vi "Earliest MultiFrameStructure Diagram UID.vi"(8 "error in (no error)":errorcluster, 11 "MFS ref in":refnum<vi>) -> (0 "error out":errorcluster, 1 "TLD?":bool, 2 "UID":i32, 3 "MFS ref out":refnum<vi>)   [LabVIEW 2019]
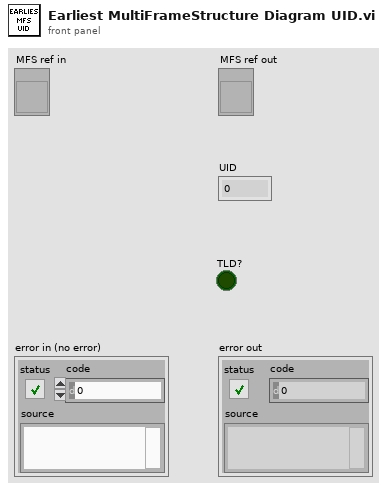
[diagram p1: front panel]
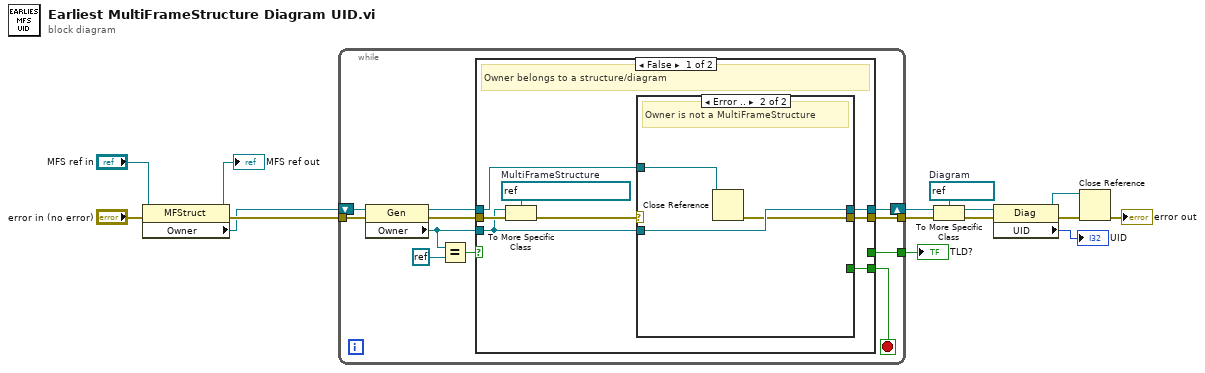
[diagram p0: block diagram]
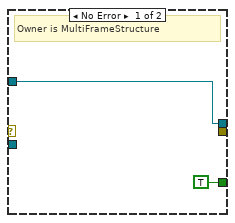
[diagram p2: hidden frame]
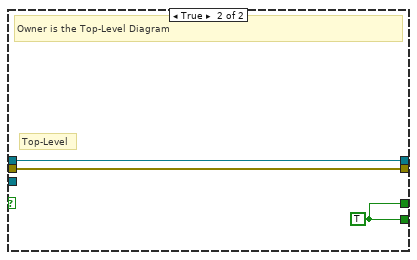
[diagram p3: hidden frame]
diagram:
  w6 = refnum<vi> refnum  # Diagram
  n1 = property class="MFStruct"(reference="MFS ref in", error in="error in (no error)") -> (reference out=→"MFS ref out":refnum<vi>, error out=w12:errorcluster, "Owner"=w11:refnum<vi>)
  n2 = while {
    tunnel: [w21] -> w7
    tunnel: w12 -> [w23]
    shift-right: [w20] -> w4
    shift-left: w11 -> [w24]
    tunnel: [w16] -> w5
    stop <- w22 stop-if-true
    n3 = property class="Gen"(reference=w24, error in=w23) -> (reference out=w17:refnum<vi>, error out=w18:errorcluster, "Owner"=w19:refnum<vi>)
    n4 = Equal?(x=w19, y=refnum<k0> refnum) -> (x = y?=w25:bool)
    n5 = case shown="False" w25 {
      tunnel: [w31 w42] -> w22
      tunnel: [_ w42] -> w21
      tunnel: [w29 w41] -> w20
      tunnel: w19 -> [w30 _]
      tunnel: w18 -> [w33 w40]
      tunnel: w17 -> [w28 w41]
      tunnel: [w27 w40] -> w16
      frame False {
        w34 = refnum<vi> refnum  # MultiFrameStructure
        # "Owner belongs to a structure/diagram"
        n6 = To More Specific Class(target class=w34, reference=w30, error in=w33) -> (error out=w32:errorcluster)  [unwired: 1 out]
        n7 = case shown="Error .." w32 {
          tunnel: [TRUE ("Boolean") _] -> w31
          tunnel: w30 -> [_ w39]
          tunnel: [w35 w39] -> w29
          tunnel: w28 -> [w35 w38]
          tunnel: [_ w37] -> w27
          frame No Error {
            # "Owner is MultiFrameStructure"
          }
          frame Error {
            # "Owner is not a MultiFrameStructure"
            n8 = Close Reference(reference=w38) -> (error out=w37:errorcluster)  [unwired: 1 in]
          }
        }
      }
      frame True {
        w42 = TRUE ("Boolean")
        # "Top-Level"
        # "Owner is the Top-Level Diagram"
      }
    }
  }
  "TLD?" <- w7
  n9 = To More Specific Class(target class=w6, reference=w4, error in=w5) -> (specific class reference=w2:refnum<vi>, error out=w3:errorcluster)
  n10 = property class="Diag"(reference=w2, error in=w3) -> (reference out=w9:refnum<vi>, error out=w10:errorcluster, "UID"=→"UID":i32)
  n11 = Close Reference(reference=w9, error in (no error)=w10) -> (error out=→"error out":errorcluster)
